vi "3.0.0_LED Test.vi"(6 ".batCMD":T1={"Brush_ADC.bat"="Brush_ADC.bat", "Get Release Version.bat"="Get Release Version.bat", "Getting Software  Version.bat"="Getting Software  Version.bat", "Pump_ADC.bat"="Pump_ADC.bat", "Starting  Pump Motor.bat"="Starting  Pump Motor.bat", "Starting  Test Mode.bat"="Starting  Test Mode.bat", "Starting Brush Motor 1.bat"="Starting Brush Motor 1.bat", "Starting Brush Motor 2.bat"="Starting Brush Motor 2.bat", "Starting Brush Motor 3.bat"="Starting Brush Motor 3.bat", "Starting LED Test.bat"="Starting LED Test.bat", "Stopping  Brush Motor.bat"="Stopping  Brush Motor.bat", "Stopping  Pump Motor.bat"="Stopping  Pump Motor.bat", "Stopping  Test Mode.bat"="Stopping  Test Mode.bat", "Starting Self Test.bat"="Starting Self Test.bat", "Software Reset.bat"="Software Reset.bat", "Get HW version.bat"="Get HW version.bat", "Read PMIC status.bat"="Read PMIC status.bat", "SC IMU Data Streaming.bat"="SC IMU Data Streaming.bat"}, 7 "Data in":T2, 8 "error in (no error)":errorcluster, 9 "AllControls In":T3, 10 "?":T4, 11 "Message Queue out":T5) -> (0 "error out":errorcluster, 1 "Flow":string, 2 "Data":T4, 3 "Message Queue Out":T5, 5 "Data out":T2)   [LabVIEW 2017]
uses:
  Depends/AMC/subVIs/TypeDefs/amc_Message Queue.ctl
  Depends/AMC/subVIs/TypeDefs/amc_Message.ctl
  Depends/Tools/Keyed Array/Tools_KeyedArray KeyedArray.ctl
  Ctrls/Data.ctl
  Ctrls/AllControls.ctl
  Ctrls/CSV_Data.ctl
  0516/X682 Chassis Connectivity Tester Program/Ctrls/682_cmd.ctl
types:
  T1 = typedef "682_cmd.ctl" = cluster{"Brush_ADC.bat":string, "Get Release Version.bat":string, "Getting Software  Version.bat":string, "Pump_ADC.bat":string, "Starting  Pump Motor.bat":string, "Starting  Test Mode.bat":string, "Starting Brush Motor 1.bat":string, "Starting Brush Motor 2.bat":string, "Starting Brush Motor 3.bat":string, "Starting LED Test.bat":string, "Stopping  Brush Motor.bat":string, "Stopping  Pump Motor.bat":string, "Stopping  Test Mode.bat":string, "Starting Self Test.bat":string, "Software Reset.bat":string, "Get HW version.bat":string, "Read PMIC status.bat":string, "SC IMU Data Streaming.bat":string}
  T2 = typedef "CSV_Data.ctl" = cluster{"Initialisation":cluster{"LMT - Connect UUT (con COM)":string, "LMT - Software Version (rrel)":string, "LMT - Write SKU file (wskuc)":string, "LMT - SKU file name":string, "Connect UUT DDM":string, "Read DDM EOL Timestamp - Mode":string, "Read DDM EOL Timestamp - Timestamp":string, "Read DDM EOL Timestamp - Rig ID":string, "Read DDM EOL Timestamp - Passmark ID":string, "Read DDM EOL Timestamp - Passmark Rev":string, "Software Version before flashing":string, "Read Hardware Serial":string, "UUT DDM SN":string, "Compare DDM SN with MES SN":string, "Backup PCBA Calibration EEPROM Response - CAL":string, "Flash Firmware Version":string, "Check SW Version":string, "Read DDM SW Version after flashing":string, "Set SKU Config":string, "Ready Status":string, "Set Device Mode to EOL":string, "DDM Parameter - Voltage":string, "DDM Parameter - Current":string, "DDM Parameter - Power":string, "DDM Parameter - Speed":string, "DDM Parameter - Pressure":string, "Tester Parameter - Voltage":string, "Tester Parameter - Current":string, "Tester Parameter - Power":string, "Tester Parameter - Ambient Pressure":string, "Tester Parameter - Ambient Temperature":string, "Calculated Parameter - DDM Pressure Corrected":string, "Calculated Parameter - DDM Real Power":string, "Calculated Parameter - Delta V":string}, "BEMF_Calibration":cluster{"Calibration Result - eol_cold_bemf_temp":string, "DDM Ambient Temp":string, "Restriction Plate Diameter":string, "Calibration Result - eol_bemf_mp_cold_coef_a":string, "Calibration Result - eol_bemf_mp_cold_coef_b":string, "Calibration Result - eol_bemf_mp_cold_coef_c":string, "Calibration Result - eol_bemf_lsi_cold_ref_coeffs":string, "Get - Calibration Result - eol_bemf_lsi_speed":string, "Get - Calibration Result - eol_bemf_lsi_integral_0":string, "Calibration Result - eol_bemf_lsi_integral_1":string, "Get - Calibration Result - eol_bemf_lsi_integral_2":string, "Get - Calibration Result - eol_cold_bemf":string, "Get - Calibration Result - eol_cold_bemf_fisf":string, "Finalise Calibration":string, "Compare -Calibration Result - eol_cold_bemf":string, "Compare -Calibration Result - eol_cold_bemf_fisf":string}, "ECO":cluster{"Reset Power Tune":string, "Reset BEMF FISF Calibration":string, "Restriction Plate Diameter":string, "ECO - Stabilisation Time":string, "ECO - DDM Parameter - Voltage":string, "ECO - DDM Parameter - Current":string, "ECO - DDM Parameter - Power":string, "ECO - DDM Parameter - Measured Power":string, "ECO - DDM Parameter - Speed":string, "ECO - DDM Parameter - Pressure":string, "ECO - Tester Parameter - Voltage":string, "ECO - Tester Parameter - Current":string, "ECO - Tester Parameter - Power":string, "ECO - Tester Parameter - Ambient Pressure":string, "ECO - Tester Parameter - Ambient Temperature":string, "ECO - Tester Parameter - Ambient Humidity":string, "ECO - Calculated Parameter - DDM Pressure Corrected":string, "ECO - Calculated Parameter - DDM Real Power":string, "ECO - Calculated Parameter - Delta V":string, "ECO - Calculated Parameter - Flowrate":string, "ECO - Calculated Parameter - Airwatt":string, "ECO - Formula":string, "PT ECO - Power Tune Mode Status":string}, "BOOST":cluster{"Restriction Plate Diameter":string, "BOOST - Stabilisation Time":string, "BOOST - DDM Parameter - Voltage":string, "BOOST - DDM Parameter - Current":string, "BOOST - DDM Parameter - Power":string, "BOOST - DDM Parameter - Measured Power":string, "BOOST - DDM Parameter - Speed":string, "BOOST - DDM Parameter - Pressure":string, "BOOST - Tester Parameter - Voltage":string, "BOOST - Tester Parameter - Current":string, "BOOST - Tester Parameter - Power":string, "BOOST - Tester Parameter - Ambient Pressure":string, "BOOST - Tester Parameter - Ambient Temperature":string, "BOOST - Tester Parameter - Ambient Humidity":string, "BOOST - Calculated Parameter - DDM Pressure Corrected":string, "BOOST - Calculated Parameter - DDM Real Power":string, "BOOST - Calculated Parameter - Delta V":string, "BOOST - Calculated Parameter - Flowrate":string, "BOOST - Calculated Parameter - Airwatt":string, "BOOST - Get AM Presence":string, "Air Muscle Turn Off Status":string, "BOOST - Air Muscle Calculated Parameter - Airwatt B":string, "BOOST - Air Muscle Calculate Airwatt Delta":string, "PT BOOST - Power Tune Mode Status":string, "Finalise Calibration":string, "ECO - Get AW Calibration value":string, "BOOST - Get AW Calibration value":string}, "MAX":cluster{"Restriction Plate Diameter":string, "MAX - Stabilisation Time":string, "Get Average Delta Tmag (LSIdelta_FISFdelta_LSItmag_FISFtmag_IIRtmag)":string, "Get Average Delta Tmag FISF":string, "MAX - DDM Parameter - Voltage":string, "MAX - DDM Parameter - Current":string, "MAX - DDM Parameter - Power":string, "MAX - DDM Parameter - Measured Power":string, "MAX - DDM Parameter - Speed":string, "MAX - DDM Parameter - Pressure":string, "MAX - Tester Parameter - Voltage":string, "MAX - Tester Parameter - Current":string, "MAX - Tester Parameter - Power":string, "MAX - Tester Parameter - Ambient Pressure":string, "MAX - Tester Parameter - Ambient Temperature":string, "MAX - Tester Parameter - Ambient Humidity":string, "MAX - Calculated Parameter - DDM Pressure Corrected":string, "MAX - Calculated Parameter - DDM Real Power":string, "MAX - Calculated Parameter - Delta V":string, "MAX - Calculated Parameter - Flowrate":string, "MAX - Calculated Parameter - Airwatt":string, "MAX_FISF_Check_Average_Delta_Tmag":string, "MAX - FISF - BEMF Finetune Result":string, "MAX tune - Delta P1":string, "MAX tune - Calculated Parameter - Airwatt":string, "Calculate Delta Airwatts - MAX finetune - Delta P2":string, "MAX finetune - DDM Parameter - Voltage":string, "MAX finetune - DDM Parameter - Current":string, "MAX finetune - DDM Parameter - Power":string, "MAX finetune - DDM Parameter - Measured Power":string, "MAX finetune - DDM Parameter - Speed":string, "MAX finetune - DDM Parameter - Pressure":string, "MAX finetune - Tester Parameter - Voltage":string, "MAX finetune - Tester Parameter - Current":string, "MAX finetune - Tester Parameter - Power":string, "MAX finetune - Tester Parameter - Ambient Pressure":string, "MAX finetune - Tester Parameter - Ambient Temperature":string, "MAX finetune - Tester Parameter - Ambient Humidity":string, "MAX finetune - Calculated Parameter - DDM Pressure Corrected":string, "MAX finetune - Calculated Parameter - DDM Real Power":string, "MAX finetune - Calculated Parameter - Delta V":string, "MAX finetune - Calculated Parameter - Flowrate":string, "MAX finetune - Calculated Parameter - Airwatt":string, "Check Derate Result":string, "Delta Tmag FISF":string, "Get Hot BEMF Result":string, "Calculate delta Pressure":string, "Finalise Calibration":string, "Calculate & Check Delta BEMF":string, "Delta P Airwatts Value":string}, "LL":cluster{"DDM Ambient Temp":string, "Restriction Plate Diameter":string, "LL - DDM Parameter - Voltage":string, "LL - DDM Parameter - Current":string, "LL - DDM Parameter - Power":string, "LL - DDM Parameter - Measured Power":string, "LL - DDM Parameter - Speed":string, "LL - DDM Parameter - Pressure":string, "LL - Tester Parameter - Voltage":string, "LL - Tester Parameter - Current":string, "LL - Tester Parameter - Power":string, "LL - DDM Real Power":string, "LL - Calibrate Task Detect LL":string}, "HL":cluster{"HL - DDM Parameter - Voltage":string, "HL - DDM Parameter - Current":string, "HL - DDM Parameter - Power":string, "HL - DDM Parameter - Measured Power":string, "HL - DDM Parameter - Speed":string, "HL - DDM Parameter - Pressure":string, "HL - Tester Parameter - Voltage":string, "HL - Tester Parameter - Current":string, "HL - Tester Parameter - Power":string, "HL - DDM Real Power":string, "HL - Calibrate Task Detect HL":string}, "LH":cluster{"Restriction Plate Diameter":string, "LH - DDM Parameter - Voltage":string, "LH - DDM Parameter - Current":string, "LH - DDM Parameter - Power":string, "LH - DDM Parameter - Measured Power":string, "LH - DDM Parameter - Speed":string, "LH - DDM Parameter - Pressure":string, "LH - Tester Parameter - Voltage":string, "LH - Tester Parameter - Current":string, "LH - Tester Parameter - Power":string, "LH - DDM Real Power":string, "LH - Calibrate Task Detect LH":string}, "HH":cluster{"HH - DDM Parameter - Voltage":string, "HH - DDM Parameter - Current":string, "HH - DDM Parameter - Power":string, "HH - DDM Parameter - Measured Power":string, "HH - DDM Parameter - Speed":string, "HH - DDM Parameter - Pressure":string, "HH - Tester Parameter - Voltage":string, "HH - Tester Parameter - Current":string, "HH - Tester Parameter - Power":string, "HH - DDM Real Power":string, "HH - Calibrate Task Detect HH":string}, "Inlet Blockage Calibration":cluster{"Inlet Blockage Calibration - DDM Parameter - Voltage":string, "Inlet Blockage Calibration - DDM Parameter - Current":string, "Inlet Blockage Calibration - DDM Parameter - Power":string, "Inlet Blockage Calibration - DDM Parameter - Measured Power":string, "Inlet Blockage Calibration - DDM Parameter - Speed":string, "Inlet Blockage Calibration - DDM Parameter - Pressure":string, "Inlet Blockage Calibration - Tester Parameter - Voltage":string, "Inlet Blockage Calibration - Tester Parameter - Current":string, "Inlet Blockage Calibration - Tester Parameter - Power":string, "Inlet Blockage Calibration - DDM Real Power":string, "Calibration Inlet Blockage_E":string, "Finalise Calibration":string, "Get Task Detect LL":string, "Get Task Detect HL":string, "Get Task Detect LH":string, "Get Task Detect HH":string, "Calibration Inlet Blockage":string, "Calibration eol cold bemf temp":string}, "GOOD":cluster{"GOOD UNIT - Clear EEPROM Error Log":string, "GOOD UNIT - Write Product Timestamp - Mode":string, "GOOD UNIT - Write Product Timestamp - Timestamp":string, "GOOD UNIT - Write Product Timestamp - Rig ID":string, "GOOD UNIT - Write Product Timestamp - Passmark ID":string, "GOOD UNIT - Write Product Timestamp - Passmark Rev":string, "GOOD UNIT - Set Device Mode to PROD":string, "GOOD UNIT - Backup PCBA Calibration EEPROM Response":string, "GOOD UNIT - Check Security Bit":string, "GOOD UNIT - Set Calibration Lock":string, "GOOD UNIT - Get_Calibration_Lock":string, "GOOD UNIT - Disconnect UUT":string}, "NG":cluster{"NG UNIT - Read NVM Error":string, "NG UNIT - Set Device Mode to FCT":string, "NG UNIT - Backup PCBA Calibration EEPROM Response - CAL":string, "NG UNIT - Backup PCBA Calibration EEPROM Response - ERROR":string, "NG UNIT - Backup PCBA Calibration EEPROM Response - USAGE":string, "NG UNIT - Disconnect UUT":string}, "SN":string, "Table":string[][], "Count":cluster{"Total":i32, "OK":i32, "NG":i32, "Yield":dbl}, "Start Time":timestamp, "daemon reference":refnum<k5>, "CT":dbl, "Config":string[][], "OK/NG":bool, "Station ID":string, "MES DDM SN":string, "MES PCBA SN":string, "Retest":string, "Lux":string, "Initialisation_Status":cluster{"LMT - Connect UUT (con COM)":string, "LMT - Software Version (rrel)":string, "LMT - Write SKU file (wskuc)":string, "LMT - SKU file name":string, "Connect UUT DDM":string, "Read DDM EOL Timestamp - Mode":string, "Read DDM EOL Timestamp - Timestamp":string, "Read DDM EOL Timestamp - Rig ID":string, "Read DDM EOL Timestamp - Passmark ID":string, "Read DDM EOL Timestamp - Passmark Rev":string, "Software Version before flashing":string, "Read Hardware Serial":string, "UUT DDM SN":string, "Compare DDM SN with MES SN":string, "Backup PCBA Calibration EEPROM Response - CAL":string, "Flash Firmware Version":string, "Check SW Version":string, "Read DDM SW Version after flashing":string, "Set SKU Config":string, "Ready Status":string, "Set Device Mode to EOL":string, "DDM Parameter - Voltage":string, "DDM Parameter - Current":string, "DDM Parameter - Power":string, "DDM Parameter - Speed":string, "DDM Parameter - Pressure":string, "Tester Parameter - Voltage":string, "Tester Parameter - Current":string, "Tester Parameter - Power":string, "Tester Parameter - Ambient Pressure":string, "Tester Parameter - Ambient Temperature":string, "Calculated Parameter - DDM Pressure Corrected":string, "Calculated Parameter - DDM Real Power":string, "Calculated Parameter - Delta V":string}, "BEMF_Calibration_Status":cluster{"Calibration Result - eol_cold_bemf_temp":string, "DDM Ambient Temp":string, "Restriction Plate Diameter":string, "Calibration Result - eol_bemf_mp_cold_coef_a":string, "Calibration Result - eol_bemf_mp_cold_coef_b":string, "Calibration Result - eol_bemf_mp_cold_coef_c":string, "Calibration Result - eol_bemf_lsi_cold_ref_coeffs":string, "Get - Calibration Result - eol_bemf_lsi_speed":string, "Get - Calibration Result - eol_bemf_lsi_integral_0":string, "Calibration Result - eol_bemf_lsi_integral_1":string, "Get - Calibration Result - eol_bemf_lsi_integral_2":string, "Get - Calibration Result - eol_cold_bemf":string, "Get - Calibration Result - eol_cold_bemf_fisf":string, "Finalise Calibration":string, "Compare -Calibration Result - eol_cold_bemf":string, "Compare -Calibration Result - eol_cold_bemf_fisf":string}, "ECO_Status":cluster{"Reset Power Tune":string, "Reset BEMF FISF Calibration":string, "Restriction Plate Diameter":string, "ECO - Stabilisation Time":string, "ECO - DDM Parameter - Voltage":string, "ECO - DDM Parameter - Current":string, "ECO - DDM Parameter - Power":string, "ECO - DDM Parameter - Measured Power":string, "ECO - DDM Parameter - Speed":string, "ECO - DDM Parameter - Pressure":string, "ECO - Tester Parameter - Voltage":string, "ECO - Tester Parameter - Current":string, "ECO - Tester Parameter - Power":string, "ECO - Tester Parameter - Ambient Pressure":string, "ECO - Tester Parameter - Ambient Temperature":string, "ECO - Tester Parameter - Ambient Humidity":string, "ECO - Calculated Parameter - DDM Pressure Corrected":string, "ECO - Calculated Parameter - DDM Real Power":string, "ECO - Calculated Parameter - Delta V":string, "ECO - Calculated Parameter - Flowrate":string, "ECO - Calculated Parameter - Airwatt":string, "ECO - Formula":string, "PT ECO - Power Tune Mode Status":string}, "BOOST_Status":cluster{"Restriction Plate Diameter":string, "BOOST - Stabilisation Time":string, "BOOST - DDM Parameter - Voltage":string, "BOOST - DDM Parameter - Current":string, "BOOST - DDM Parameter - Power":string, "BOOST - DDM Parameter - Measured Power":string, "BOOST - DDM Parameter - Speed":string, "BOOST - DDM Parameter - Pressure":string, "BOOST - Tester Parameter - Voltage":string, "BOOST - Tester Parameter - Current":string, "BOOST - Tester Parameter - Power":string, "BOOST - Tester Parameter - Ambient Pressure":string, "BOOST - Tester Parameter - Ambient Temperature":string, "BOOST - Tester Parameter - Ambient Humidity":string, "BOOST - Calculated Parameter - DDM Pressure Corrected":string, "BOOST - Calculated Parameter - DDM Real Power":string, "BOOST - Calculated Parameter - Delta V":string, "BOOST - Calculated Parameter - Flowrate":string, "BOOST - Calculated Parameter - Airwatt":string, "BOOST - Get AM Presence":string, "Air Muscle Turn Off Status":string, "BOOST - Air Muscle Calculated Parameter - Airwatt B":string, "BOOST - Air Muscle Calculate Airwatt Delta":string, "PT BOOST - Power Tune Mode Status":string, "Finalise Calibration":string, "ECO - Get AW Calibration value":string, "BOOST - Get AW Calibration value":string}, "MAX_Status":cluster{"Restriction Plate Diameter":string, "MAX - Stabilisation Time":string, "Get Average Delta Tmag (LSIdelta_FISFdelta_LSItmag_FISFtmag_IIRtmag)":string, "Get Average Delta Tmag FISF":string, "MAX - DDM Parameter - Voltage":string, "MAX - DDM Parameter - Current":string, "MAX - DDM Parameter - Power":string, "MAX - DDM Parameter - Measured Power":string, "MAX - DDM Parameter - Speed":string, "MAX - DDM Parameter - Pressure":string, "MAX - Tester Parameter - Voltage":string, "MAX - Tester Parameter - Current":string, "MAX - Tester Parameter - Power":string, "MAX - Tester Parameter - Ambient Pressure":string, "MAX - Tester Parameter - Ambient Temperature":string, "MAX - Tester Parameter - Ambient Humidity":string, "MAX - Calculated Parameter - DDM Pressure Corrected":string, "MAX - Calculated Parameter - DDM Real Power":string, "MAX - Calculated Parameter - Delta V":string, "MAX - Calculated Parameter - Flowrate":string, "MAX - Calculated Parameter - Airwatt":string, "MAX_FISF_Check_Average_Delta_Tmag":string, "MAX - FISF - BEMF Finetune Result":string, "MAX tune - Delta P1":string, "MAX tune - Calculated Parameter - Airwatt":string, "Calculate Delta Airwatts - MAX finetune - Delta P2":string, "MAX finetune - DDM Parameter - Voltage":string, "MAX finetune - DDM Parameter - Current":string, "MAX finetune - DDM Parameter - Power":string, "MAX finetune - DDM Parameter - Measured Power":string, "MAX finetune - DDM Parameter - Speed":string, "MAX finetune - DDM Parameter - Pressure":string, "MAX finetune - Tester Parameter - Voltage":string, "MAX finetune - Tester Parameter - Current":string, "MAX finetune - Tester Parameter - Power":string, "MAX finetune - Tester Parameter - Ambient Pressure":string, "MAX finetune - Tester Parameter - Ambient Temperature":string, "MAX finetune - Tester Parameter - Ambient Humidity":string, "MAX finetune - Calculated Parameter - DDM Pressure Corrected":string, "MAX finetune - Calculated Parameter - DDM Real Power":string, "MAX finetune - Calculated Parameter - Delta V":string, "MAX finetune - Calculated Parameter - Flowrate":string, "MAX finetune - Calculated Parameter - Airwatt":string, "Check Derate Result":string, "Delta Tmag FISF":string, "Get Hot BEMF Result":string, "Calculate delta Pressure":string, "Finalise Calibration":string, "Calculate & Check Delta BEMF":string, "Delta P Airwatts Value":string}, "LL_Status":cluster{"DDM Ambient Temp":string, "Restriction Plate Diameter":string, "LL - DDM Parameter - Voltage":string, "LL - DDM Parameter - Current":string, "LL - DDM Parameter - Power":string, "LL - DDM Parameter - Measured Power":string, "LL - DDM Parameter - Speed":string, "LL - DDM Parameter - Pressure":string, "LL - Tester Parameter - Voltage":string, "LL - Tester Parameter - Current":string, "LL - Tester Parameter - Power":string, "LL - DDM Real Power":string, "LL - Calibrate Task Detect LL":string}, "HL_Status":cluster{"HL - DDM Parameter - Voltage":string, "HL - DDM Parameter - Current":string, "HL - DDM Parameter - Power":string, "HL - DDM Parameter - Measured Power":string, "HL - DDM Parameter - Speed":string, "HL - DDM Parameter - Pressure":string, "HL - Tester Parameter - Voltage":string, "HL - Tester Parameter - Current":string, "HL - Tester Parameter - Power":string, "HL - DDM Real Power":string, "HL - Calibrate Task Detect HL":string}, "LH_Status":cluster{"Restriction Plate Diameter":string, "LH - DDM Parameter - Voltage":string, "LH - DDM Parameter - Current":string, "LH - DDM Parameter - Power":string, "LH - DDM Parameter - Measured Power":string, "LH - DDM Parameter - Speed":string, "LH - DDM Parameter - Pressure":string, "LH - Tester Parameter - Voltage":string, "LH - Tester Parameter - Current":string, "LH - Tester Parameter - Power":string, "LH - DDM Real Power":string, "LH - Calibrate Task Detect LH":string}, "HH_Status":cluster{"HH - DDM Parameter - Voltage":string, "HH - DDM Parameter - Current":string, "HH - DDM Parameter - Power":string, "HH - DDM Parameter - Measured Power":string, "HH - DDM Parameter - Speed":string, "HH - DDM Parameter - Pressure":string, "HH - Tester Parameter - Voltage":string, "HH - Tester Parameter - Current":string, "HH - Tester Parameter - Power":string, "HH - DDM Real Power":string, "HH - Calibrate Task Detect HH":string}, "Inlet Blockage Calibration_Status":cluster{"Inlet Blockage Calibration - DDM Parameter - Voltage":string, "Inlet Blockage Calibration - DDM Parameter - Current":string, "Inlet Blockage Calibration - DDM Parameter - Power":string, "Inlet Blockage Calibration - DDM Parameter - Measured Power":string, "Inlet Blockage Calibration - DDM Parameter - Speed":string, "Inlet Blockage Calibration - DDM Parameter - Pressure":string, "Inlet Blockage Calibration - Tester Parameter - Voltage":string, "Inlet Blockage Calibration - Tester Parameter - Current":string, "Inlet Blockage Calibration - Tester Parameter - Power":string, "Inlet Blockage Calibration - DDM Real Power":string, "Calibration Inlet Blockage_E":string, "Finalise Calibration":string, "Get Task Detect LL":string, "Get Task Detect HL":string, "Get Task Detect LH":string, "Get Task Detect HH":string, "Calibration Inlet Blockage":string, "Calibration eol cold bemf temp":string}, "GOOD_Status":cluster{"GOOD UNIT - Clear EEPROM Error Log":string, "GOOD UNIT - Write Product Timestamp - Mode":string, "GOOD UNIT - Write Product Timestamp - Timestamp":string, "GOOD UNIT - Write Product Timestamp - Rig ID":string, "GOOD UNIT - Write Product Timestamp - Passmark ID":string, "GOOD UNIT - Write Product Timestamp - Passmark Rev":string, "GOOD UNIT - Set Device Mode to PROD":string, "GOOD UNIT - Backup PCBA Calibration EEPROM Response":string, "GOOD UNIT - Check Security Bit":string, "GOOD UNIT - Set Calibration Lock":string, "GOOD UNIT - Get_Calibration_Lock":string, "GOOD UNIT - Disconnect UUT":string}, "NG_Status":cluster{"NG UNIT - Read NVM Error":string, "NG UNIT - Set Device Mode to FCT":string, "NG UNIT - Backup PCBA Calibration EEPROM Response - CAL":string, "NG UNIT - Backup PCBA Calibration EEPROM Response - ERROR":string, "NG UNIT - Backup PCBA Calibration EEPROM Response - USAGE":string, "NG UNIT - Disconnect UUT":string}, "SKU":string, "Plate_Diameter":string, "Alarm":string}
  T3 = typedef "AllControls.ctl" = cluster{"MainVI":refnum<vi>, "AlarmInfo":refnum<vi>, "Log":refnum<vi>, "Current CT":refnum<vi>, "ProductID":refnum<vi>, "Device state":refnum<vi>, "MES":refnum<vi>, "mode":refnum<vi>, "TestInfo":refnum<vi>, "SubPnl":refnum<vi>, "Table":refnum<vi>, "MES bool":refnum<vi>, "TestMode":refnum<vi>, "Recipe":refnum<vi>, "Fail resume":refnum<vi>, "LogIn":refnum<vi>, "Start":refnum<vi>, "Maintenance":refnum<vi>, "Stop":refnum<vi>, "Exit":refnum<vi>}
  T4 = typedef "Data.ctl" = cluster{"Initialisation":cluster{"DDM_Parameter":dbl[], "DDM_Parameter_status":bool[], "Get_Tester_Parameter":dbl[], "Get_Tester_Parameter_status":bool[], "Cal_Tester_Parameter":dbl[], "Cal_Tester_Parameter_status":bool[], "sw_version_before_status":bool, "sw_version_after_status":bool, "Set_SKU_Config_With_LMT_status":bool, "FCT_timestamp_status":bool, "LMT_Connect_to_UUT_status":bool}, "BEMF_Calibration":cluster{"Read_ambient_temperature":dbl, "Calibration_Vaule":dbl[], "Calibration_Vaule _B":dbl[], "Calibration_Vaule_status":bool[], "Calibration_Vaule_B_status":bool[]}, "ECO":cluster{"DDM_Parameter":dbl[], "DDM_Parameter_status":bool[], "Get_Tester_Parameter":dbl[], "Get_Tester_Parameter_status":bool[], "Cal_Tester_Parameter":dbl[], "Cal_Tester_Parameter_status":bool[], "DDM_Parameter_after_power_tune":dbl[], "Get_Tester_Parameter_after_power_tune":dbl[], "Cal_Tester_Parameter_after_power_tune":dbl[], "Cal_Tester_Parameter_after_power_tune_status":bool[], "Delta_P":dbl}, "BOOST":cluster{"DDM_Parameter":dbl[], "DDM_Parameter_status":bool[], "Get_Tester_Parameter":dbl[], "Get_Tester_Parameter_status":bool[], "Cal_Tester_Parameter":dbl[], "Cal_Tester_Parameter_status":bool[], "DDM_Parameter_after_power_tune":dbl[], "Get_Tester_Parameter_after_power_tune":dbl[], "Cal_Tester_Parameter_after_power_tune":dbl[], "Cal_Tester_Parameter_after_power_tune_status":bool[], "airwatts_am_off":dbl, "AW_Delta_(AM_on_and_off)":dbl, "AW_Delta_(AM_on_and_off)_Status":bool, "Delta_P":dbl}, "MAX":cluster{"Average_Tmag_Data":cluster{"LSI Delta in degC":dbl, "FISF Delta in degc":dbl, "LSI Tmag in degC":dbl, "Fisf Tmag in degC":dbl, "IIR Tmag in degC":dbl}, "DDM_Parameter":dbl[], "DDM_Parameter_status":bool[], "Get_Tester_Parameter":dbl[], "Get_Tester_Parameter_status":bool[], "Cal_Tester_Parameter":dbl[], "BEMF_Finetune":cluster{"eol_bemf_mp_cold_coef_c":dbl, "eol_cold_bemf_fisf_offset":dbl}, "AW_Tune":cluster{"delta_P1":dbl, "delta_P_Setting":dbl}, "DDM_Parameter_after_Airwatts_Tune":dbl[], "Get_Tester_Parameter_after_Airwatts_Tune":dbl[], "Cal_Tester_Parameter_after_Airwatts_Tune":dbl[], "DDM_Parameter_after_Airwatts_Finetune":dbl[], "Get_Tester_Parameter_after_Airwatts_Finetune":dbl[], "Cal_Tester_Parameter_after_Airwatts_Finetune":dbl[], "AW_Finetune":cluster{"delta_P2":dbl, "delta_P_Setting":dbl}, "Delta_Tmag_after_tune":cluster{"LSI Delta in degC":dbl, "FISF Delta in degc":dbl, "LSI Tmag in degC":dbl, "Fisf Tmag in degC":dbl, "IIR Tmag in degC":dbl}, "Hot Bemf in mV":dbl, "DDM_Pressure":dbl, "Delta_Pressure":dbl, " Cold Bemf in mV":dbl, " delta Bemf":dbl, " delta p":dbl, "Delta_Pressure_status":bool, " delta Bemf_status":bool, "LSI Delta in degC_status":bool, "FISF Delta in degc_status":bool, "Max_check_derate_status_status":bool, "Average_All_data":dbl[][], "Average_Tmag_Data_status":bool[], "Average_Tmag_Data_after_tune_status":bool[], "Cal_Tester_Parameter_status":bool[], "Cal_Tester_Parameter_status_after_Airwatts_Tune":bool[], "Cal_Tester_Parameter_status_after_Airwatts_FineTune":bool[]}, "Task_Detect_Calib":cluster{"LL":cluster{"DDM_Parameter":dbl[], "DDM_Parameter_status":bool[], "Get_Tester_Parameter":dbl[], "Get_Tester_Parameter_status":bool[], "Set_task_detect_A":dbl, "Set_task_detect_A_Status":bool}, "HL":cluster{"DDM_Parameter":dbl[], "DDM_Parameter_status":bool[], "Get_Tester_Parameter":dbl[], "Get_Tester_Parameter_status":bool[], "Set_task_detect_B":dbl, "Set_task_detect_B_Status":bool}, "LH":cluster{"DDM_Parameter":dbl[], "DDM_Parameter_status":bool[], "Get_Tester_Parameter":dbl[], "Get_Tester_Parameter_status":bool[], "Set_task_detect_C":dbl, "Set_task_detect_C_Status":bool}, "HH":cluster{"DDM_Parameter":dbl[], "DDM_Parameter_status":bool[], "Get_Tester_Parameter":dbl[], "Get_Tester_Parameter_status":bool[], "Set_task_detect_D":dbl, "Read_and_check_calibration_Status":bool[], "Set_task_detect_D_Status":bool}, "Get_eol_inlet_blockage_E":dbl, "Calib_vaule":cluster{"Get_task_detect_LL":dbl, "Get_task_detect_HL":dbl, "Get_task_detect_LH":dbl, "Get_task_detect_HH":dbl, "eol_inlet_blockage":dbl, "eol_code_bemf_temp":dbl}, "calibrated temp":dbl, "Inlet_Blockage_Calibration":cluster{"DDM_Parameter":dbl[], "DDM_Parameter_status":bool[], "Get_Tester_Parameter":dbl[], "Get_Tester_Parameter_status":bool[]}, "Get_eol_inlet_blockage_E_Status":bool}, "good":cluster{"Write_Product_TS":cluster{"TIMESTAMP":i64, "RIG_ID":i64, "PASSMARK_ID":i64, "PASSMARK_REV":i64}, "Read_Product_TS":cluster{"TIMESTAMP":i64, "RIG_ID":i64, "PASSMARK_ID":i64, "PASSMARK_REV":i64}, "Good_Check_Secuity_Bit_Stauts":bool}}
  T5 = typedef "amc_Message Queue.ctl" = refnum<queue>
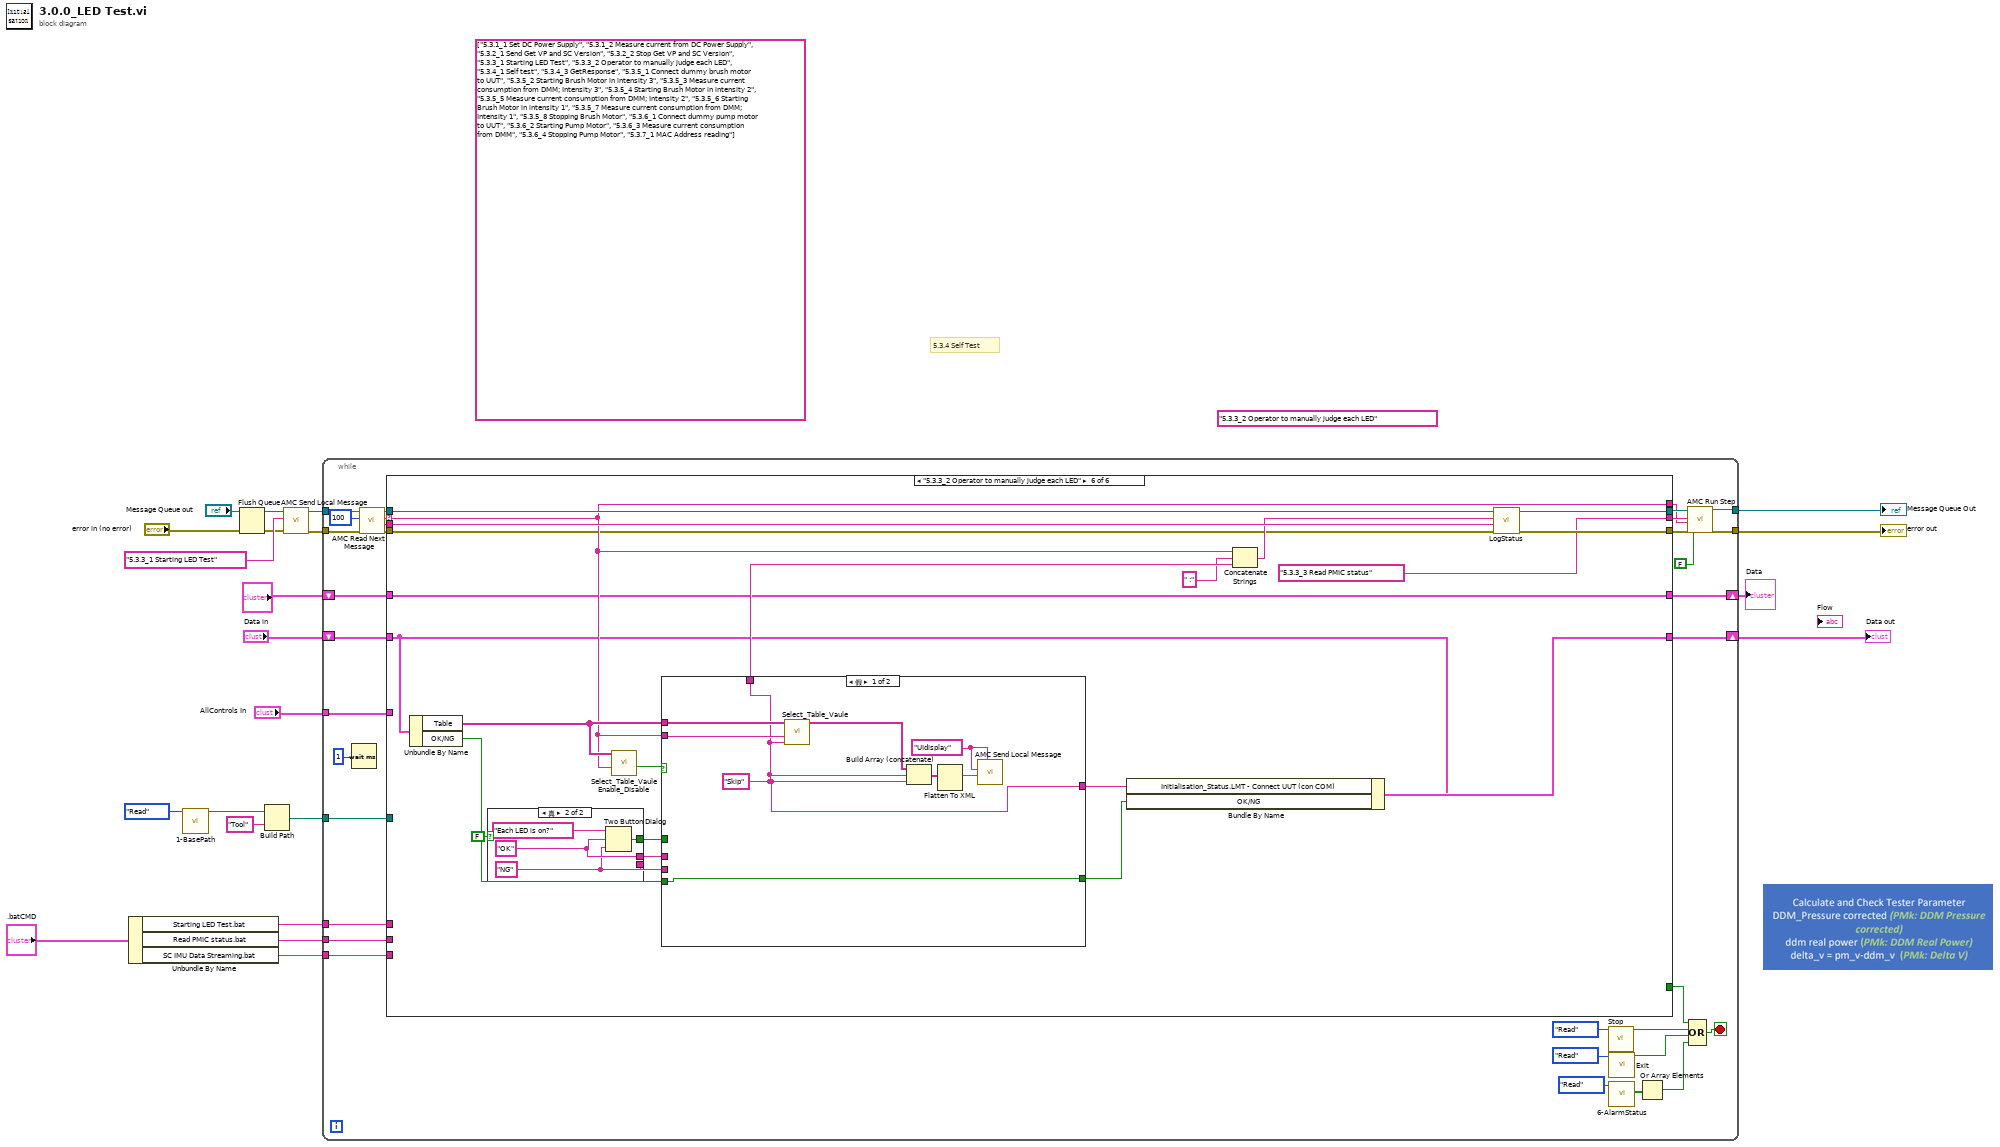
[diagram p0: block diagram]
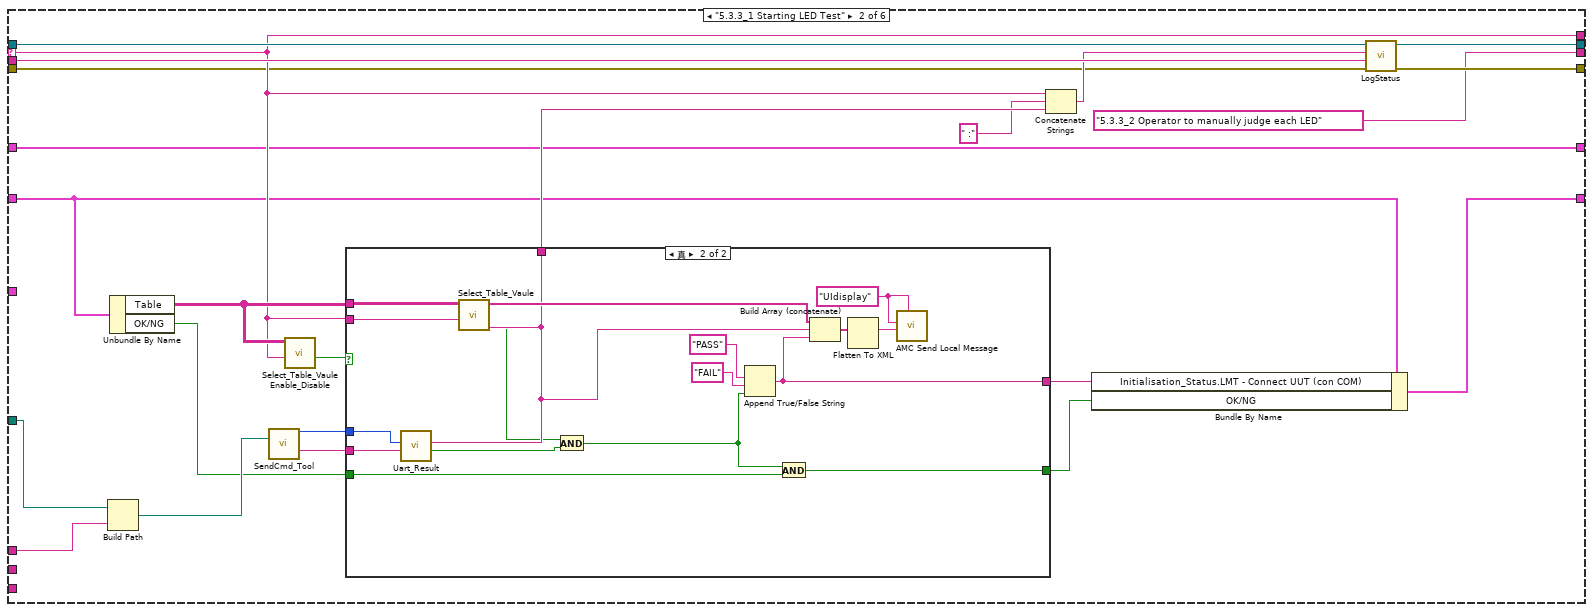
[diagram p3: hidden frame]
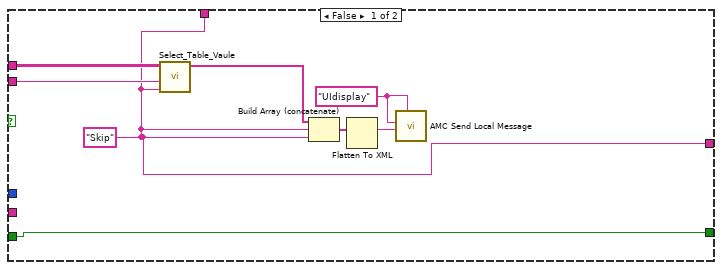
[diagram p4: hidden frame]
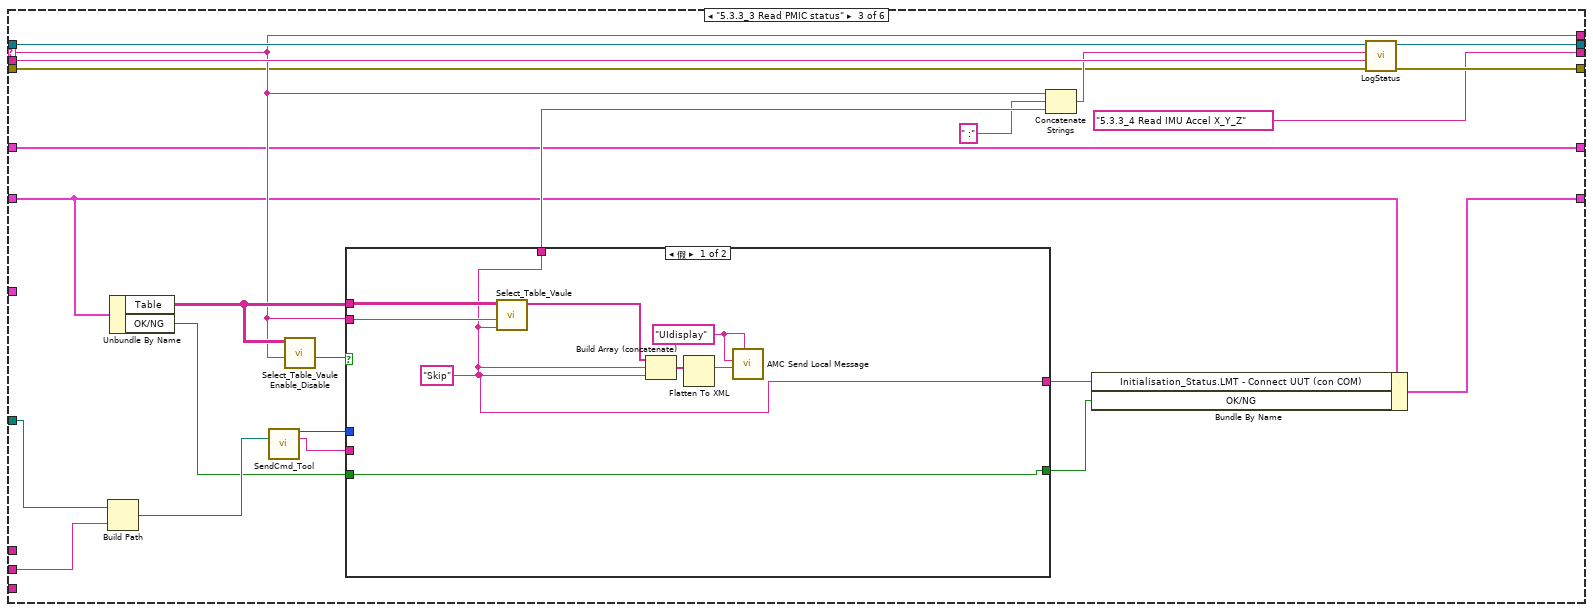
[diagram p5: hidden frame]
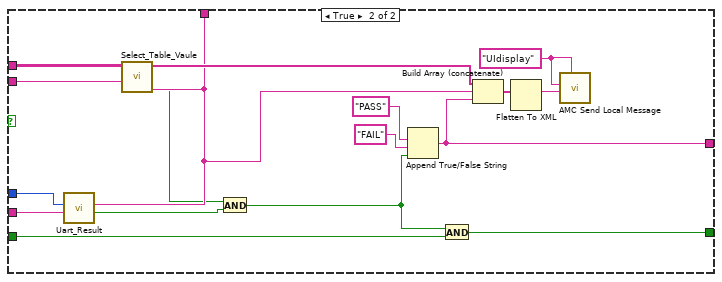
[diagram p6: hidden frame]
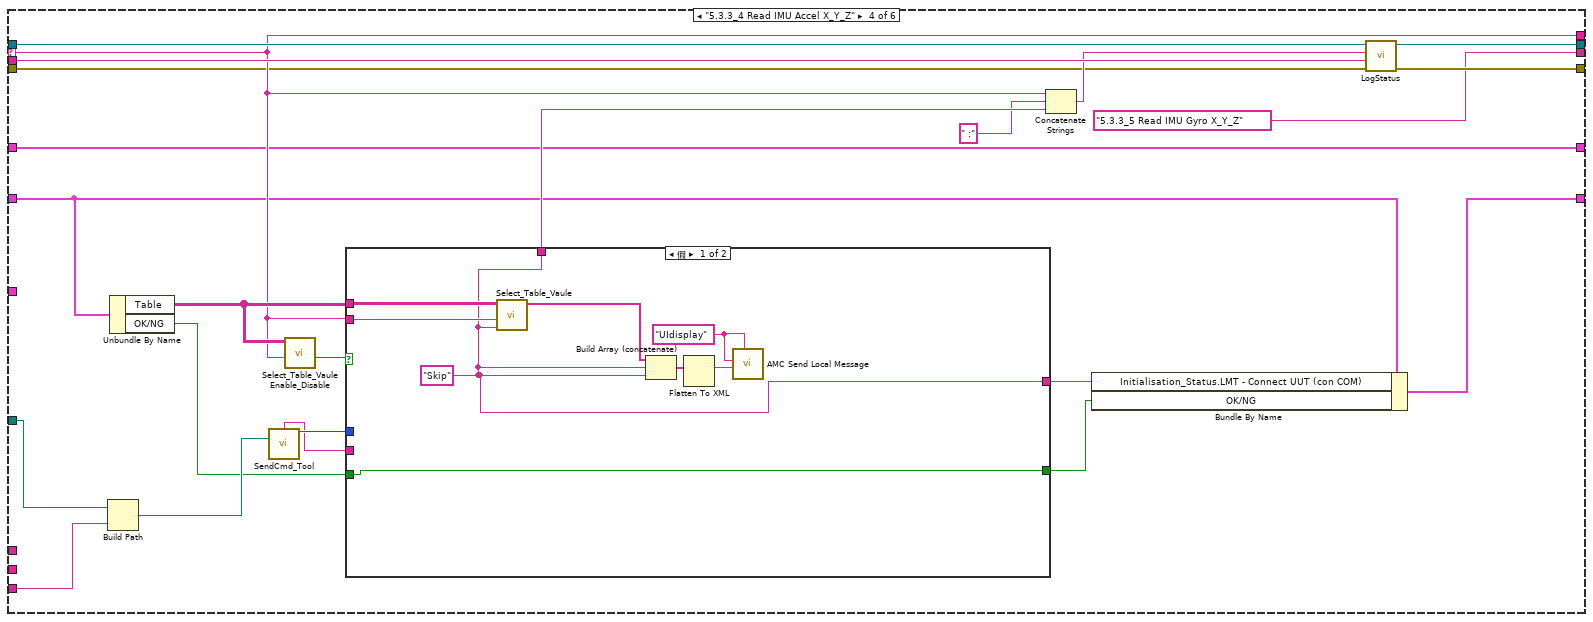
[diagram p7: hidden frame]
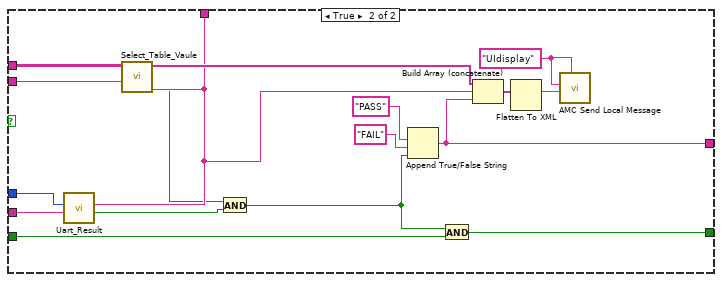
[diagram p8: hidden frame]
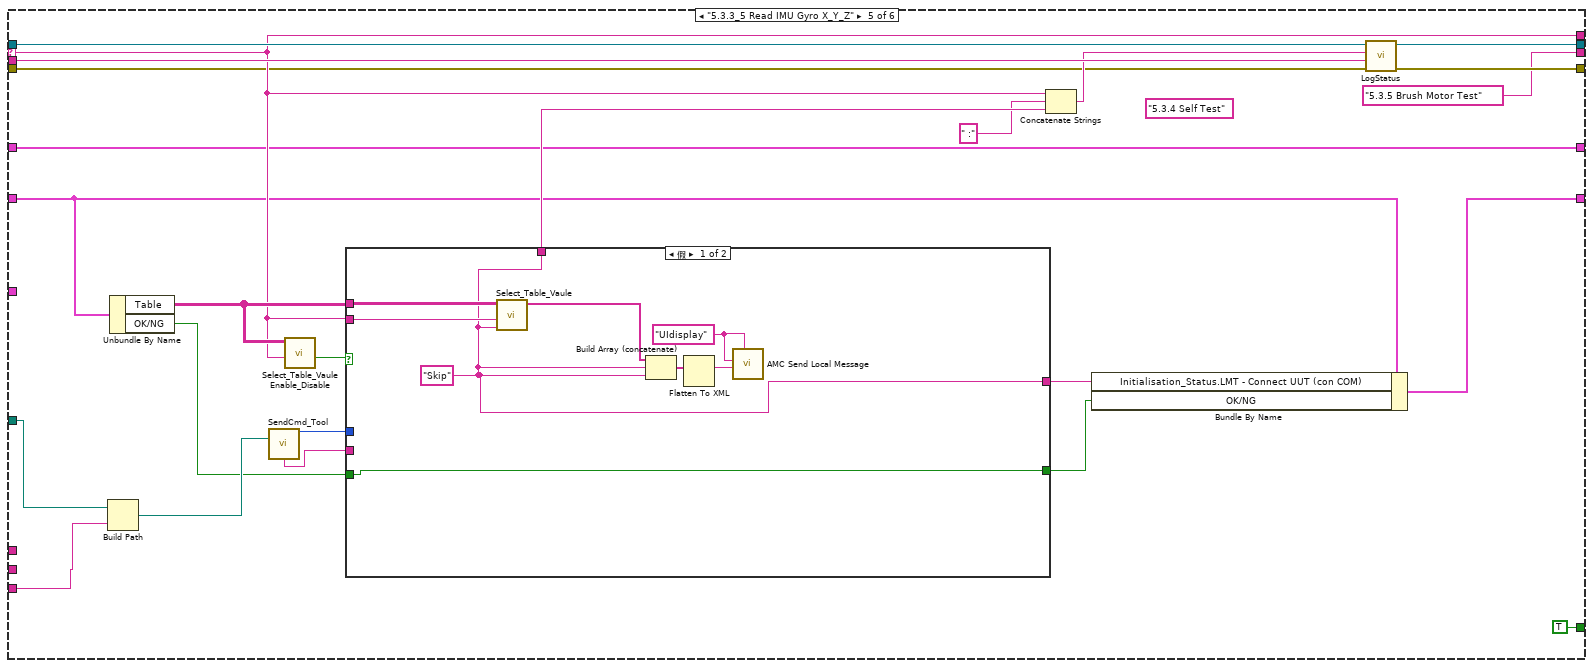
[diagram p9: hidden frame]
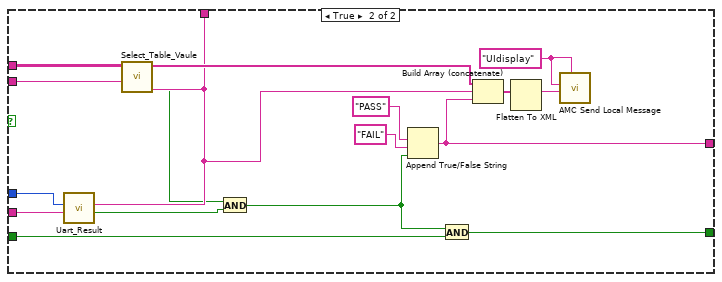
[diagram p10: hidden frame]
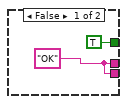
[diagram p11: hidden frame]
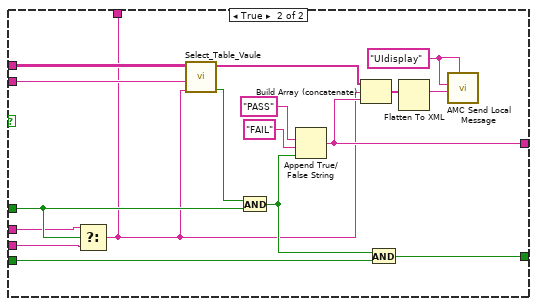
[diagram p12: hidden frame]
diagram:
  (unwired) "5.3.3_2 Operator to manually judge each LED"
  (unwired) string[] ["5.3.1_1 Set DC Power Supply", "5.3.1_2 Measure current from DC Power Supply", "5.3.2_1 Send Get VP and SC Version", "5.3.2_2 Stop Get VP and SC Version", "5.3.3_1 Starting LED Test", "5.3.3_2 Operator to manually judge each LED", "5.3.4_1 Self test", "5.3.4_3 GetResponse", "5.3.5_1 Connect dummy brush motor to UUT", "5.3.5_2 Starting Brush Motor in intensity 3", "5.3.5_3 Measure current consumption from DMM; Intensity 3", "5.3.5_4 Starting Brush Motor in intensity 2", "5.3.5_5 Measure current consumption from DMM; Intensity 2", "5.3.5_6 Starting Brush Motor in intensity 1", "5.3.5_7 Measure current consumption from DMM; Intensity 1", "5.3.5_8 Stopping Brush Motor", "5.3.6_1 Connect dummy pump motor to UUT", "5.3.6_2 Starting Pump Motor", "5.3.6_3 Measure current consumption from DMM", "5.3.6_4 Stopping Pump Motor", "5.3.7_1 MAC Address reading"] ("subarray")
  # "5.3.4 Self Test"
  n1 = Unbundle By Name(".batCMD") -> ("Starting LED Test.bat"=w4:string, "Read PMIC status.bat"=w3:string, "SC IMU Data Streaming.bat"=w1:string)
  n2 = call "1-BasePath.vi"("Step"=enum16{"Initial", "Write", "Read"}."Read") -> ("Path Out"=w6:path)  [unwired: 9 in, 1 out]
  n3 = Flush Queue(queue="Message Queue out") -> (queue out=w14:T5)  [unwired: 1 in, 2 out]
  n4 = Build Path(base path=w6, name or relative path="Tool") -> (appended path=w5:path)
  n5 = call "AMC Send Local Message.vi"("error in (no error)"="error in (no error)", "Message Name"="5.3.3_1 Starting LED Test", "Message Queue in"=w14) -> ("error out"=w18:errorcluster, "Message Queue out"=w19:T5)  [unwired: 7 in]
  n6 = while {
    tunnel: w19 -> [w54]
    tunnel: [w50] -> w13
    tunnel: w18 -> [w48]
    tunnel: [w45] -> w12
    shift-right: [w41] -> w15
    shift-left: "?" -> [w42]
    tunnel: "AllControls In" -> [w31]
    shift-right: [w29] -> w9
    shift-left: "Data in" -> [w30]
    tunnel: w5 -> [w25]
    tunnel: w4 -> [w24]
    tunnel: w3 -> [w23]
    tunnel: w1 -> [w22]
    stop <- w34 stop-if-true
    n7 = Wait (ms)(milliseconds to wait=u32 1 ("等待时间（毫秒）")) -> ()  [unwired: 1 out]
    n8 = call "AMC Read Next Message.vi"("error in (no error)"=w48, "timeout (1ms)"=100, "Message Queue in"=w54) -> ("error out"=w47:errorcluster, "Message Value"=w39:string, "Message Name"=w52:string, "Message Queue out"=w53:T5)  [unwired: 1 in, 4 out]
    n9 = case shown="\"5.3.3_2 Operator to manually judge each LED\"" w52 {
      selector: w52 -> [_ w75 w122 w169 w217 w263]
      tunnel: w53 -> [w58 w80 w127 w174 w222 w268]
      tunnel: [w58 w80 w127 w174 w222 w268] -> w51
      tunnel: w47 -> [w57 w74 w121 w168 w216 w262]
      tunnel: [w57 w79 w126 w173 w221 w267] -> w46
      tunnel: [_ _ _ _ TRUE ("GRR") _] -> w35
      tunnel: w42 -> [w56 w70 w117 w164 w213 w258]
      tunnel: [w56 w70 w117 w164 w213 w258] -> w41
      tunnel: w39 -> [_ w78 w125 w172 w220 w266]
      tunnel: [_ w75 w122 w169 w217 w263] -> w38
      tunnel: [_ "5.3.3_2 Operator to manually judge each LED" "5.3.3_4 Read IMU Accel X_Y_Z" "5.3.3_5 Read IMU Gyro X_Y_Z" "5.3.5 Brush Motor Test" "5.3.3_3 Read PMIC status"] -> w40
      tunnel: w31 -> [_ _ _ _ _ _]
      tunnel: w30 -> [w55 w69 w116 w163 w212 w248]
      tunnel: [w55 w68 w115 w162 w211 w257] -> w29
      tunnel: w25 -> [_ w65 w113 w160 w208 _]
      tunnel: w24 -> [_ w59 _ _ _ _]
      tunnel: w23 -> [_ _ w112 _ _ _]
      tunnel: w22 -> [_ _ _ w154 w200 _]
      frame "假", Default {
      }
      frame "5.3.3_1 Starting LED Test" {
        n10 = Build Path(base path=w65, name or relative path=w59) -> (appended path=w64:path)
        n11 = Unbundle By Name(w69) -> ("Table"=w76:string[][], "OK/NG"=w62:bool)
        n12 = call "SendCmd_Tool.vi"("path_bat"=w64) -> ("return code"=w63:i32, "Led Test"=w66:string)  [unwired: 6 in, 7 out]
        n13 = call "Select_Table_Vaule Enable_Disable.vi"("Action"=w75, "Table"=w76) -> ("Enable"=w72:bool)  [unwired: 8 in, 1 out]
        n14 = case shown="真" w72 {
          tunnel: [w82 w91] -> w73
          tunnel: w76 -> [w84 w99]
          tunnel: w75 -> [w83 w98]
          tunnel: w66 -> [_ w92]
          tunnel: [w82 w97] -> w67
          tunnel: w63 -> [_ w93]
          tunnel: w62 -> [w81 w95]
          tunnel: [w81 w94] -> w61
          frame False {
            w88 = "UIdisplay" ("Process (\"\" - local)")
            w82 = "Skip" ("Action")
            n15 = call "Select_Table_Vaule.vi"("Vaule"=w82, "Action"=w83, "Table"=w84) -> ("vaule"=w85:string[])  [unwired: 7 in, 1 out]
            n16 = Build Array (concatenate)(w85, w82, w82) -> (w87:string[])
            n17 = Flatten To XML(anything=w87) -> (xml string=w86:string)
            n18 = call "AMC Send Local Message.vi"("Process (\"\" - local)"=w88, "Message Value"=w86, "Message Name"=w88) -> ()  [unwired: 7 in, 2 out]
          }
          frame True {
            w104 = "UIdisplay" ("Process (\"\" - local)")
            n19 = call "Uart_Result.vi"("input"=w92, "return code"=w93) -> ("Command Sucess"=w89:bool, "return_result"=w91:string)  [unwired: 8 in]
            n20 = call "Select_Table_Vaule.vi"("Vaule"=w91, "Action"=w98, "Table"=w99) -> ("Result"=w90:bool, "vaule"=w105:string[])  [unwired: 7 in]
            n21 = And(x=w90, y=w89) -> (x .and. y?=w96:bool)
            n22 = Append True/False String(1:w96, 2:"FAIL" ("真字符串"), 3:"PASS" ("真字符串")) -> (0:w97:string)  [unwired: 1 in]
            n23 = And(x=w96, y=w95) -> (x .and. y?=w94:bool)
            n24 = Build Array (concatenate)(w105, w91, w97) -> (w103:string[])
            n25 = Flatten To XML(anything=w103) -> (xml string=w102:string)
            n26 = call "AMC Send Local Message.vi"("Process (\"\" - local)"=w104, "Message Value"=w102, "Message Name"=w104) -> ()  [unwired: 7 in, 2 out]
          }
        }
        n27 = Concatenate Strings(w75, " :", w73) -> (w77:string)
        n28 = Bundle By Name(cluster=w69, "Initialisation_Status.LMT - Connect UUT (con COM)"=w67, "OK/NG"=w61) -> (w68:T2)
        n29 = call "LogStatus.vi"("error in (no error)"=w74, "last message"=w78, "message"=w77) -> ("error  out"=w79:errorcluster)  [unwired: 8 in]
      }
      frame "5.3.3_3 Read PMIC status" {
        n30 = Build Path(base path=w113, name or relative path=w112) -> (appended path=w111:path)
        n31 = Unbundle By Name(w116) -> ("Table"=w123:string[][], "OK/NG"=w109:bool)
        n32 = call "SendCmd_Tool.vi"("path_bat"=w111) -> ("return code"=w110:i32, "Other"=w106:string)  [unwired: 6 in, 7 out]
        n33 = call "Select_Table_Vaule Enable_Disable.vi"("Action"=w122, "Table"=w123) -> ("Enable"=w119:bool)  [unwired: 8 in, 1 out]
        n34 = case shown="假" w119 {
          tunnel: [w129 w138] -> w120
          tunnel: w123 -> [w131 w146]
          tunnel: w122 -> [w130 w145]
          tunnel: w106 -> [_ w139]
          tunnel: [w129 w144] -> w114
          tunnel: w110 -> [_ w140]
          tunnel: w109 -> [w128 w142]
          tunnel: [w128 w141] -> w108
          frame False {
            w135 = "UIdisplay" ("Process (\"\" - local)")
            w129 = "Skip" ("Action")
            n35 = call "Select_Table_Vaule.vi"("Vaule"=w129, "Action"=w130, "Table"=w131) -> ("vaule"=w132:string[])  [unwired: 7 in, 1 out]
            n36 = Build Array (concatenate)(w132, w129, w129) -> (w134:string[])
            n37 = Flatten To XML(anything=w134) -> (xml string=w133:string)
            n38 = call "AMC Send Local Message.vi"("Process (\"\" - local)"=w135, "Message Value"=w133, "Message Name"=w135) -> ()  [unwired: 7 in, 2 out]
          }
          frame True {
            w151 = "UIdisplay" ("Process (\"\" - local)")
            n39 = call "Uart_Result.vi"("input"=w139, "return code"=w140) -> ("Command Sucess"=w136:bool, "return_result"=w138:string)  [unwired: 8 in]
            n40 = call "Select_Table_Vaule.vi"("Vaule"=w138, "Action"=w145, "Table"=w146) -> ("Result"=w137:bool, "vaule"=w152:string[])  [unwired: 7 in]
            n41 = And(x=w137, y=w136) -> (x .and. y?=w143:bool)
            n42 = Append True/False String(1:w143, 2:"FAIL" ("真字符串"), 3:"PASS" ("真字符串")) -> (0:w144:string)  [unwired: 1 in]
            n43 = And(x=w143, y=w142) -> (x .and. y?=w141:bool)
            n44 = Build Array (concatenate)(w152, w138, w144) -> (w150:string[])
            n45 = Flatten To XML(anything=w150) -> (xml string=w149:string)
            n46 = call "AMC Send Local Message.vi"("Process (\"\" - local)"=w151, "Message Value"=w149, "Message Name"=w151) -> ()  [unwired: 7 in, 2 out]
          }
        }
        n47 = Concatenate Strings(w122, " :", w120) -> (w124:string)
        n48 = Bundle By Name(cluster=w116, "Initialisation_Status.LMT - Connect UUT (con COM)"=w114, "OK/NG"=w108) -> (w115:T2)
        n49 = call "LogStatus.vi"("error in (no error)"=w121, "last message"=w125, "message"=w124) -> ("error  out"=w126:errorcluster)  [unwired: 8 in]
      }
      frame "5.3.3_4 Read IMU Accel X_Y_Z" {
        n50 = Build Path(base path=w160, name or relative path=w154) -> (appended path=w159:path)
        n51 = Unbundle By Name(w163) -> ("Table"=w170:string[][], "OK/NG"=w157:bool)
        n52 = call "SendCmd_Tool.vi"("path_bat"=w159) -> ("Accel_XYZ"=w153:string, "return code"=w158:i32)  [unwired: 6 in, 7 out]
        n53 = call "Select_Table_Vaule Enable_Disable.vi"("Action"=w169, "Table"=w170) -> ("Enable"=w166:bool)  [unwired: 8 in, 1 out]
        n54 = case shown="假" w166 {
          tunnel: [w176 w185] -> w167
          tunnel: w170 -> [w178 w193]
          tunnel: w169 -> [w177 w192]
          tunnel: w153 -> [_ w186]
          tunnel: [w176 w191] -> w161
          tunnel: w158 -> [_ w187]
          tunnel: w157 -> [w175 w189]
          tunnel: [w175 w188] -> w156
          frame False {
            w182 = "UIdisplay" ("Process (\"\" - local)")
            w176 = "Skip" ("Action")
            n55 = call "Select_Table_Vaule.vi"("Vaule"=w176, "Action"=w177, "Table"=w178) -> ("vaule"=w179:string[])  [unwired: 7 in, 1 out]
            n56 = Build Array (concatenate)(w179, w176, w176) -> (w181:string[])
            n57 = Flatten To XML(anything=w181) -> (xml string=w180:string)
            n58 = call "AMC Send Local Message.vi"("Process (\"\" - local)"=w182, "Message Value"=w180, "Message Name"=w182) -> ()  [unwired: 7 in, 2 out]
          }
          frame True {
            w198 = "UIdisplay" ("Process (\"\" - local)")
            n59 = call "Uart_Result.vi"("input"=w186, "return code"=w187) -> ("Command Sucess"=w183:bool, "return_result"=w185:string)  [unwired: 8 in]
            n60 = call "Select_Table_Vaule.vi"("Vaule"=w185, "Action"=w192, "Table"=w193) -> ("Result"=w184:bool, "vaule"=w199:string[])  [unwired: 7 in]
            n61 = And(x=w184, y=w183) -> (x .and. y?=w190:bool)
            n62 = Append True/False String(1:w190, 2:"FAIL" ("真字符串"), 3:"PASS" ("真字符串")) -> (0:w191:string)  [unwired: 1 in]
            n63 = And(x=w190, y=w189) -> (x .and. y?=w188:bool)
            n64 = Build Array (concatenate)(w199, w185, w191) -> (w197:string[])
            n65 = Flatten To XML(anything=w197) -> (xml string=w196:string)
            n66 = call "AMC Send Local Message.vi"("Process (\"\" - local)"=w198, "Message Value"=w196, "Message Name"=w198) -> ()  [unwired: 7 in, 2 out]
          }
        }
        n67 = Concatenate Strings(w169, " :", w167) -> (w171:string)
        n68 = Bundle By Name(cluster=w163, "Initialisation_Status.LMT - Connect UUT (con COM)"=w161, "OK/NG"=w156) -> (w162:T2)
        n69 = call "LogStatus.vi"("error in (no error)"=w168, "last message"=w172, "message"=w171) -> ("error  out"=w173:errorcluster)  [unwired: 8 in]
      }
      frame "5.3.3_5 Read IMU Gyro X_Y_Z" {
        (unwired) "5.3.4 Self Test"
        n70 = Build Path(base path=w208, name or relative path=w200) -> (appended path=w207:path)
        n71 = Unbundle By Name(w212) -> ("Table"=w218:string[][], "OK/NG"=w205:bool)
        n72 = call "SendCmd_Tool.vi"("path_bat"=w207) -> ("return code"=w206:i32, "Gyro_XYZ"=w201:string)  [unwired: 6 in, 7 out]
        n73 = call "Select_Table_Vaule Enable_Disable.vi"("Action"=w217, "Table"=w218) -> ("Enable"=w214:bool)  [unwired: 8 in, 1 out]
        n74 = case shown="假" w214 {
          tunnel: [w224 w233] -> w215
          tunnel: w218 -> [w226 w241]
          tunnel: w217 -> [w225 w240]
          tunnel: w201 -> [_ w234]
          tunnel: [w224 w239] -> w210
          tunnel: w206 -> [_ w235]
          tunnel: w205 -> [w223 w237]
          tunnel: [w223 w236] -> w204
          frame False {
            w230 = "UIdisplay" ("Process (\"\" - local)")
            w224 = "Skip" ("Action")
            n75 = call "Select_Table_Vaule.vi"("Vaule"=w224, "Action"=w225, "Table"=w226) -> ("vaule"=w227:string[])  [unwired: 7 in, 1 out]
            n76 = Build Array (concatenate)(w227, w224, w224) -> (w229:string[])
            n77 = Flatten To XML(anything=w229) -> (xml string=w228:string)
            n78 = call "AMC Send Local Message.vi"("Process (\"\" - local)"=w230, "Message Value"=w228, "Message Name"=w230) -> ()  [unwired: 7 in, 2 out]
          }
          frame True {
            w246 = "UIdisplay" ("Process (\"\" - local)")
            n79 = call "Uart_Result.vi"("input"=w234, "return code"=w235) -> ("Command Sucess"=w231:bool, "return_result"=w233:string)  [unwired: 8 in]
            n80 = call "Select_Table_Vaule.vi"("Vaule"=w233, "Action"=w240, "Table"=w241) -> ("Result"=w232:bool, "vaule"=w247:string[])  [unwired: 7 in]
            n81 = And(x=w232, y=w231) -> (x .and. y?=w238:bool)
            n82 = Append True/False String(1:w238, 2:"FAIL" ("真字符串"), 3:"PASS" ("真字符串")) -> (0:w239:string)  [unwired: 1 in]
            n83 = And(x=w238, y=w237) -> (x .and. y?=w236:bool)
            n84 = Build Array (concatenate)(w247, w233, w239) -> (w245:string[])
            n85 = Flatten To XML(anything=w245) -> (xml string=w244:string)
            n86 = call "AMC Send Local Message.vi"("Process (\"\" - local)"=w246, "Message Value"=w244, "Message Name"=w246) -> ()  [unwired: 7 in, 2 out]
          }
        }
        n87 = Concatenate Strings(w217, " :", w215) -> (w219:string)
        n88 = Bundle By Name(cluster=w212, "Initialisation_Status.LMT - Connect UUT (con COM)"=w210, "OK/NG"=w204) -> (w211:T2)
        n89 = call "LogStatus.vi"("error in (no error)"=w216, "last message"=w220, "message"=w219) -> ("error  out"=w221:errorcluster)  [unwired: 8 in]
      }
      frame "5.3.3_2 Operator to manually judge each LED" {
        n90 = Unbundle By Name(w248) -> ("Table"=w264:string[][], "OK/NG"=w253:bool)
        n91 = case shown="真" FALSE {
          tunnel: [TRUE ("T button?") w273] -> w255
          tunnel: [w269 w272] -> w252
          tunnel: [w269 w271] -> w251
          frame False {
            w269 = "OK" ("T按钮名称（“确定”）")
          }
          frame True {
            w271 = "NG" ("F按钮名称（“取消”）")
            w272 = "OK" ("T按钮名称（“确定”）")
            n92 = Two Button Dialog(message="Each LED is on?" ("消息"), 1:w271, 2:w272) -> (T button?=w273:bool)
          }
        }
        n93 = call "Select_Table_Vaule Enable_Disable.vi"("Action"=w263, "Table"=w264) -> ("Enable"=w260:bool)  [unwired: 8 in, 1 out]
        n94 = case shown="假" w260 {
          tunnel: [w276 w283] -> w261
          tunnel: w264 -> [w278 w293]
          tunnel: w263 -> [w277 w292]
          tunnel: [w276 w291] -> w256
          tunnel: w255 -> [_ w286]
          tunnel: w253 -> [w275 w288]
          tunnel: [w275 w287] -> w254
          tunnel: w252 -> [_ w285]
          tunnel: w251 -> [_ w284]
          frame False {
            w282 = "UIdisplay" ("Process (\"\" - local)")
            w276 = "Skip" ("Action")
            n95 = call "Select_Table_Vaule.vi"("Vaule"=w276, "Action"=w277, "Table"=w278) -> ("vaule"=w279:string[])  [unwired: 7 in, 1 out]
            n96 = Build Array (concatenate)(w279, w276, w276) -> (w281:string[])
            n97 = Flatten To XML(anything=w281) -> (xml string=w280:string)
            n98 = call "AMC Send Local Message.vi"("Process (\"\" - local)"=w282, "Message Value"=w280, "Message Name"=w282) -> ()  [unwired: 7 in, 2 out]
          }
          frame True {
            w298 = "UIdisplay" ("Process (\"\" - local)")
            n99 = Select(t=w285, s=w286, f=w284) -> (s? t:f=w283:string)
            n100 = call "Select_Table_Vaule.vi"("Vaule"=w283, "Action"=w292, "Table"=w293) -> ("Result"=w290:bool, "vaule"=w299:string[])  [unwired: 7 in]
            n101 = And(x=w290, y=w286) -> (x .and. y?=w289:bool)
            n102 = Append True/False String(1:w289, 2:"FAIL" ("真字符串"), 3:"PASS" ("真字符串")) -> (0:w291:string)  [unwired: 1 in]
            n103 = Build Array (concatenate)(w299, w283, w291) -> (w297:string[])
            n104 = And(x=w289, y=w288) -> (x .and. y?=w287:bool)
            n105 = Flatten To XML(anything=w297) -> (xml string=w296:string)
            n106 = call "AMC Send Local Message.vi"("Process (\"\" - local)"=w298, "Message Value"=w296, "Message Name"=w298) -> ()  [unwired: 7 in, 2 out]
          }
        }
        n107 = Bundle By Name(cluster=w248, "Initialisation_Status.LMT - Connect UUT (con COM)"=w256, "OK/NG"=w254) -> (w257:T2)
        n108 = Concatenate Strings(w263, " :", w261) -> (w265:string)
        n109 = call "LogStatus.vi"("error in (no error)"=w262, "last message"=w266, "message"=w265) -> ("error  out"=w267:errorcluster)  [unwired: 8 in]
      }
    }
    n110 = call "Stop.vi"("Step"=enum16{"Initial", "Write", "Read"}."Read") -> ("Stop Out"=w33:bool)  [unwired: 9 in, 1 out]
    n111 = call "Exit.vi"("Step"=enum16{"Initial", "Write", "Read"}."Read" ("step")) -> ("Exit Out"=w32:bool)  [unwired: 9 in, 1 out]
    n112 = call "6-AlarmStatus.vi"("Step"=enum16{"Initial", "Write", "Read"}."Read") -> ("AlarmValue Out"=w27:bool[])  [unwired: 9 in, 1 out]
    n113 = Or Array Elements(Boolean array=w27) -> (logical OR=w26:bool)
    n114 = call "AMC Run Step.vi"("Message Queue In"=w51, "Message Name"=w40, "Message Value"=w38, "error in (no error)"=w46, "Mli/Sig"=FALSE) -> ("Message Queue Out"=w50:T5, "error out"=w45:errorcluster)  [unwired: 13 in]
    n115 = Compound Arithmetic op=OR(w35, w33, w32, w26) -> (w34:bool)
  }
  "Message Queue Out" <- w13
  "error out" <- w12
  "Data" <- w15
  "Data out" <- w9
